vi "post_dust_event_small.vi"(8 "error in (no error)":errorcluster, 10 "Signal Array":T1[](array[typedef]), 11 "Cluster":T4 {"File Location" items=["Unknown"=-1, "Storage"=0, "Processing"=1]}) -> (0 "error out":errorcluster, 1 "Experiment Settings":i32, 2 "Dust Event ID":i64)   [LabVIEW 2013]
uses:
  <vilib>/addons/database/_DB Variant To Data/Database Variant To Data.xnode
  NaN_screening_small.vi
  User Interface/Controls/File_location.ctl
  User Interface/Controls/Hardware ID.ctl
  User Interface/Controls/Role ID.ctl
  User Interface/Controls/Signal.ctl
  User Interface/Controls/Post_Dust_Event_small.ctl
panel:
  # "Signal"
  # "Dust Event Small"
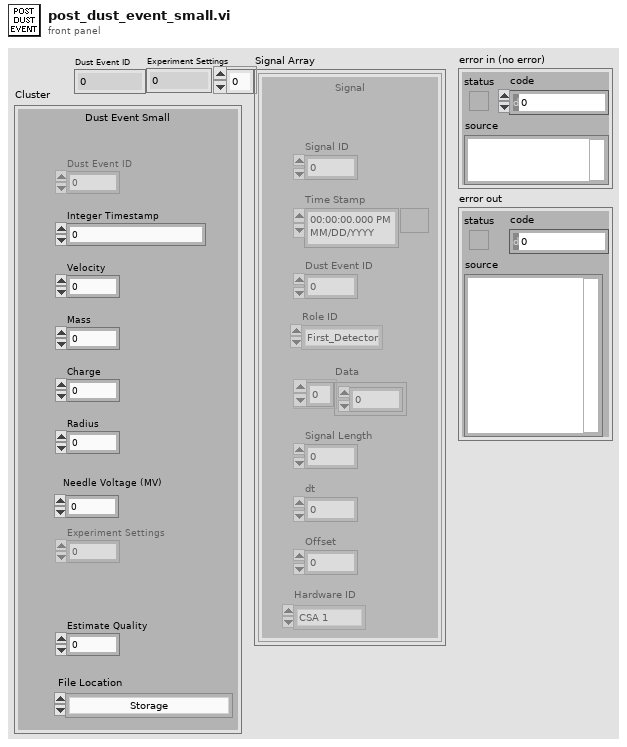
[diagram p1: front panel]
types:
  T1 = typedef "Signal.ctl" = cluster{"Signal ID":i64, "Time Stamp":timestamp, "Dust Event ID":i64, "Role ID":T2, "Data":sgl[], "Signal Length":i32, "dt":sgl, "Offset":dbl, "Hardware ID":T3}
  T2 = typedef "Role ID.ctl" = enum16{"First_Detector", "Second_Detector", "Third_Detector", "LeCroy_CH1", "LeCroy_CH2", "LeCroy_CH3", "LeCroy_CH4", "PSU", "DCS 1", "DCS 2"}
  T3 = typedef "Hardware ID.ctl" = enum16{"Unknown", "CSA 1", "CSA 2", "CSA 3", "CSA 4", "CSA 5", "CSA 6", "DCS 1", "DCS 2"}
  T4 = typedef "Post_Dust_Event_small.ctl" = cluster{"Dust Event ID":i64, "Integer Timestamp":i64, "Velocity":sgl, "Mass":sgl, "Charge":sgl, "Radius":sgl, "Needle Voltage (MV)":dbl, "Experiment Settings":dbl, "Estimate Quality":sgl, "File Location":T5, "id_dust_info":dbl}
  T5 = typedef "File_location.ctl" = i8
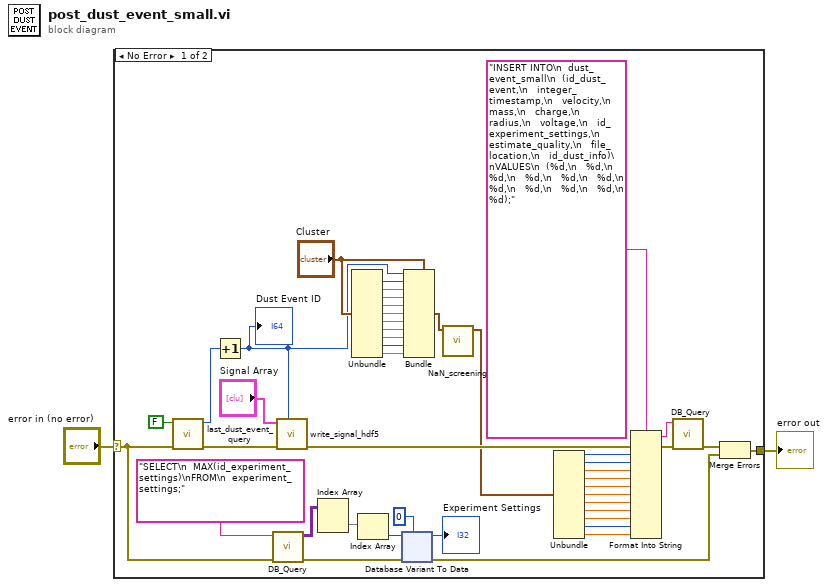
[diagram p0: block diagram]
diagram:
  n1 = case shown="No Error" "error in (no error)" {
    selector: "error in (no error)" -> [w24 w79]
    tunnel: [w46 w79] -> w1
    frame No Error {
      n2 = call "last_dust_event_query.vi"("error in (no error)"=w24, "Small?"=FALSE) -> ("error out"=w30:errorcluster, "id_dust_event"=w29:i64)  [unwired: 8 in]
      n3 = Increment(x=w29) -> (x+1=w33:i64)
      "Dust Event ID" <- w33
      n4 = call "DB_Query.vi"("error in (no error)"=w24, "Parameterized Query"="SELECT\n  MAX(id_experiment_settings)\nFROM\n  experiment_settings;" ("SQL query")) -> ("error out"=w27:errorcluster, "Results"=w25:variant[][])  [unwired: 7 in, 1 out]
      n5 = call "write_signal_hdf5.vi"("Index"=w33, "error in"=w30, "Signal array"="Signal Array") -> ("error out"=w17:errorcluster)  [unwired: 7 in, 1 out]
      n6 = Index Array(array=w25) -> (element=w21:variant[])  [unwired: 2 in]
      n7 = Unbundle("Cluster") -> ("Integer Timestamp"=w34:i64, "Velocity"=w35:sgl, "Mass"=w36:sgl, "Charge"=w37:sgl, "Radius"=w38:sgl, "Needle Voltage (MV)"=w39:dbl, "Experiment Settings"=w40:dbl, "Estimate Quality"=w41:sgl, "File Location"=w32:T5, "id_dust_info"=w42:dbl)  [unwired: 1 out]
      n8 = Index Array(array=w21) -> (element=w20:variant)  [unwired: 1 in]
      n9 = xnode "Database Variant To Data"("database variant"=w20, "error in (no error)"=w27, "type"=0) -> ("data"=→"Experiment Settings":i32, "error out"=w26:errorcluster)
      n10 = Bundle(cluster="Cluster", "Dust Event ID"=w33, "Integer Timestamp"=w34, "Velocity"=w35, "Mass"=w36, "Charge"=w37, "Radius"=w38, "Needle Voltage (MV)"=w39, "Experiment Settings"=w40, "Estimate Quality"=w41, "File Location"=w32, "id_dust_info"=w42) -> (w43:T4)
      n11 = call-poly "NaN_screening.vi"("Input"=w43) -> ("Output"=w14:T4)  [unwired: 10 in]
      n12 = Unbundle(w14) -> ("Dust Event ID"=w13:i64, "Integer Timestamp"=w3:i64, "Velocity"=w4:sgl, "Mass"=w5:sgl, "Charge"=w6:sgl, "Radius"=w7:sgl, "Needle Voltage (MV)"=w8:dbl, "Experiment Settings"=w9:dbl, "Estimate Quality"=w10:sgl, "File Location"=w11:T5, "id_dust_info"=w12:dbl)
      n13 = Format Into String(format string="INSERT INTO\n  dust_event_small\n  (id_dust_event,\n   integer_timestamp,\n   velocity,\n   mass,\n   charge,\n   radius,\n   voltage,\n   id_experiment_settings,\n   estimate_quality,\n   file_location,\n   id_dust_info)\nVALUES\n  (%d,\n   %d,\n   %d,\n   %d,\n   %d,\n   %d,\n   %d,\n   %d,\n   %d,\n   %d,\n   %d);" ("Parameterized Query"), error in=w17, w13, w3, w4, w5, w6, w7, w8, w9, w10, w11, w12) -> (resulting string=w15:string, error out=w16:errorcluster)  [unwired: 1 in]
      n14 = call "DB_Query.vi"("error in (no error)"=w16, "Parameterized Query"=w15) -> ("error out"=w19:errorcluster)  [unwired: 7 in, 2 out]
      n15 = Merge Errors(w19, w26) -> (w46:errorcluster)
    }
    frame Error {
    }
  }
  "error out" <- w1
